vi "GVISA Mux Set Path.vi"(8 "error in":errorcluster, 9 "path tag (empty)":string, 10 "path index (0: default)":i32, 11 "session in":T1={"VISA"="", "paths"=[], "idn command"="", "serial cfg"={"Baud rate"=9600, "Data bits"=8, "Parity"=0, "Stop bits"=10, "Flow control"=0, "End Mode Read"=enum."None", "End Mode Write"=enum."None", "Term character"=0, "Term enable"=FALSE}} {"serial cfg"."Flow control" items=["None", "XON/XOFF", "CTS/RTS", "XON/XOFF + CTS/RTS", "DTR/DSR", "XON/XOFF + DTR/DSR"]; "serial cfg"."Stop bits" items=["1 bit"=10, "1.5 bits"=15, "2 bits"=20]; "serial cfg"."Parity" items=["None", "Odd", "Even", "Mark", "Space"]; "serial cfg"."Data bits" items=["5 bits"=5, "6 bits"=6, "7 bits"=7, "8 bits"=8]; "serial cfg"."Baud rate" items=["150 Bd"=150, "300 Bd"=300, "600 Bd"=600, "1200 Bd"=1200, "2400 Bd"=2400, "4800 Bd"=4800, "9600 Bd"=9600, "19.2 kBd"=19200, "38.4 kBd"=38400, "57.6 kBd"=57600, "115.2 kBd"=115200]}) -> (0 "error out":errorcluster, 2 "path tag":string, 3 "session out":T1={"VISA"="", "paths"=[], "idn command"="", "serial cfg"={"Baud rate"=9600, "Data bits"=8, "Parity"=0, "Stop bits"=10, "Flow control"=0, "End Mode Read"=enum."None", "End Mode Write"=enum."None", "Term character"=0, "Term enable"=FALSE}} {"serial cfg"."Flow control" items=["None", "XON/XOFF", "CTS/RTS", "XON/XOFF + CTS/RTS", "DTR/DSR", "XON/XOFF + DTR/DSR"]; "serial cfg"."Stop bits" items=["1 bit"=10, "1.5 bits"=15, "2 bits"=20]; "serial cfg"."Parity" items=["None", "Odd", "Even", "Mark", "Space"]; "serial cfg"."Data bits" items=["5 bits"=5, "6 bits"=6, "7 bits"=7, "8 bits"=8]; "serial cfg"."Baud rate" items=["150 Bd"=150, "300 Bd"=300, "600 Bd"=600, "1200 Bd"=1200, "2400 Bd"=2400, "4800 Bd"=4800, "9600 Bd"=9600, "19.2 kBd"=19200, "38.4 kBd"=38400, "57.6 kBd"=57600, "115.2 kBd"=115200]})   [LabVIEW 2020]
doc: "Set path of generic VISA command mutiplexer. Path is defined either by 0-based index or tag string (case-sensitive). Tag string has preference over path index."
uses:
  GVISA Mux Session.ctl
  GVISA Mux Path Entry.ctl
  met_serial_setup.ctl
  <vilib>/Utility/error.llb/Error Cluster From Error Code.vi
  <vilib>/ErrorRing/Error Ring.xnode
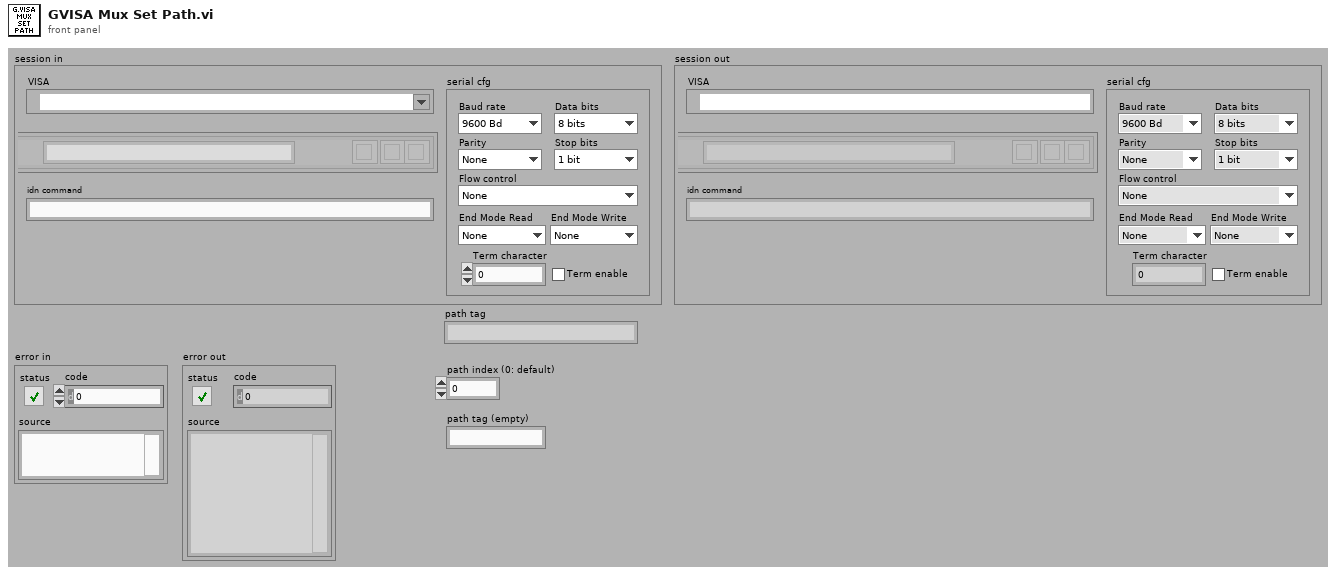
[diagram p1: front panel]
types:
  T1 = typedef "GVISA Mux Session.ctl" = cluster{"VISA":refnum<visa-resource-name>, "paths":T2[], "idn command":string, "serial cfg":T3}
  T2 = typedef "GVISA Mux Path Entry.ctl" = cluster{"Tag:":string, "Command:":string, "btn clr":bool, "btn up":bool, "btn down":bool}
  T3 = typedef "met_serial_setup.ctl" = cluster{"Baud rate":i32, "Data bits":i32, "Parity":i32, "Stop bits":i32, "Flow control":i32, "End Mode Read":enum16{"None", "Last Bit", "TermChar"}, "End Mode Write":enum16{"None", "Last Bit", "TermChar"}, "Term character":u8, "Term enable":bool}
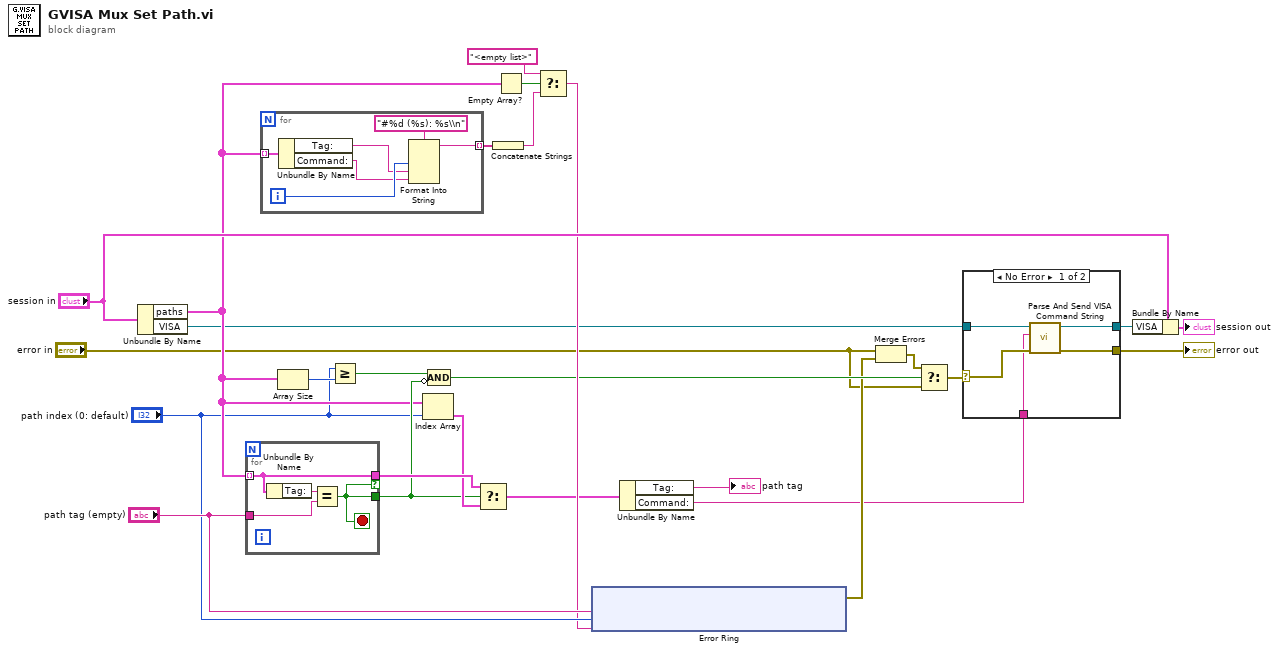
[diagram p0: block diagram]
diagram:
  n1 = Unbundle By Name("session in") -> ("paths"=w18:T2[], "VISA"=w5:refnum<visa-resource-name>)
  n2 = for {
    tunnel: w18 -> [w29] mode=indexing
    tunnel: "path tag (empty)" -> [w30]
    tunnel: [w29] -> w24 if=w27
    tunnel: [w27] -> w20
    stop <- w27 stop-if-true
    n3 = Unbundle By Name(w29) -> ("Tag:"=w28:string)
    n4 = Equal?(x=w28, y=w30) -> (x = y?=w27:bool)
  }
  n5 = for {
    tunnel: w18 -> [w36] mode=indexing
    tunnel: [w31] -> w19 mode=indexing
    i -> [w34]
    n6 = Unbundle By Name(w36) -> ("Tag:"=w33:string, "Command:"=w32:string)
    n7 = Format Into String(format string="#%d (%s): %s\\n", w34, w33, w32) -> (resulting string=w31:string)  [unwired: 2 in, 1 out]
  }
  n8 = Array Size(array=w18) -> (size(s)=w22:i32)
  n9 = Greater Or Equal?(x="path index (0: default)", y=w22) -> (x >= y?=w21:bool)
  n10 = Index Array(array=w18, index="path index (0: default)") -> (element=w23:T2)
  n11 = Compound Arithmetic op=AND(w21, invert w20) -> (w11:bool)
  n12 = Select(t=w24, s=w20, f=w23) -> (s? t:f=w4:T2)
  n13 = Concatenate Strings(w19) -> (w16:string)
  n14 = Empty Array?(array=w18) -> (empty?=w17:bool)
  n15 = Select(t="<empty list>", s=w17, f=w16) -> (s? t:f=w12:string)
  n16 = xnode "Error Ring"("parameter 0"="path tag (empty)", "parameter 1"="path index (0: default)", "parameter 2"=w12) -> ("error out"=w10:errorcluster)
  n17 = Unbundle By Name(w4) -> ("Tag:"=→"path tag":string, "Command:"=w3:string)
  n18 = Merge Errors("error in", w10) -> (w9:errorcluster)
  n19 = Select(t=w9, s=w11, f="error in") -> (s? t:f=w8:errorcluster)
  n20 = case shown="No Error" w8 {
    selector: w8 -> [w40 w42]
    tunnel: [w41 w42] -> w6
    tunnel: w5 -> [w39 w43]
    tunnel: w3 -> [w38 _]
    tunnel: [w37 w43] -> w1
    frame No Error {
      n21 = call "Parse And Send VISA Command String.vi"("error in"=w40, "command"=w38, "VISA in"=w39) -> ("error out"=w41:errorcluster, "VISA out"=w37:refnum<visa-resource-name>)  [unwired: 6 in, 1 out]
    }
    frame Error {
    }
  }
  "error out" <- w6
  n22 = Bundle By Name(cluster="session in", "VISA"=w1) -> (→"session out":T1)
